vi "SetTriggerDelay.vi"(8 "error in (no error)":errorcluster, 10 "Arg":string, 11 "PCO in":refnum<class "PCO_Camera.lvclass">) -> (0 "error out":errorcluster, 2 "setValue out":dbl, 3 "PCO out":refnum<class "PCO_Camera.lvclass">)   [LabVIEW 2020, in "PCO_Camera.lvclass"]
uses:
  PCO_Camera.lvclass
  PCO_Camera.lvclass/PCO_Camera.ctl
  pco.labview/pco.camera/Camera.lvclass
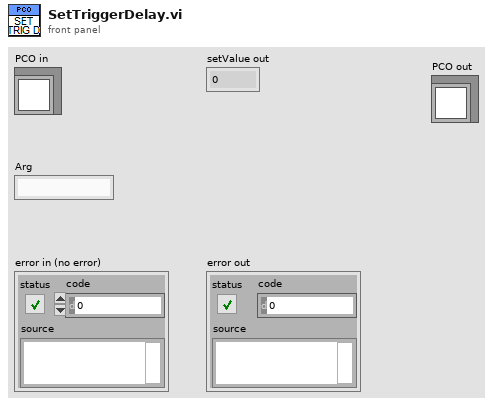
[diagram p1: front panel]
types:
  T1 = enum16{"sequence", "sequence non blocking", "ring buffer", "fifo", "sequence_dpcore", "sequence_non_blocking_dpcore", "ring_buffer_dpcore", "fifo_dpcore", "tif", "multitif", "pcoraw", "b16", "dicom", "multidicom"}
  T2 = typedef "Camera.lvclass/binning.ctl" = cluster{"vert":u16, "horz":u16}
  T3 = cluster{"exposure_time_s":dbl, "delay_time_s":dbl, "roi":cluster{"x0":u64, "y0":u64, "x1":u64, "y1":u64}, "timestamp_mode":u16, "pixelrate":u32, "trigger_mode":u16, "acquire_mode":u16, "metadata_mode":u16, "noisefilter_mode":u16, "binning":T2}
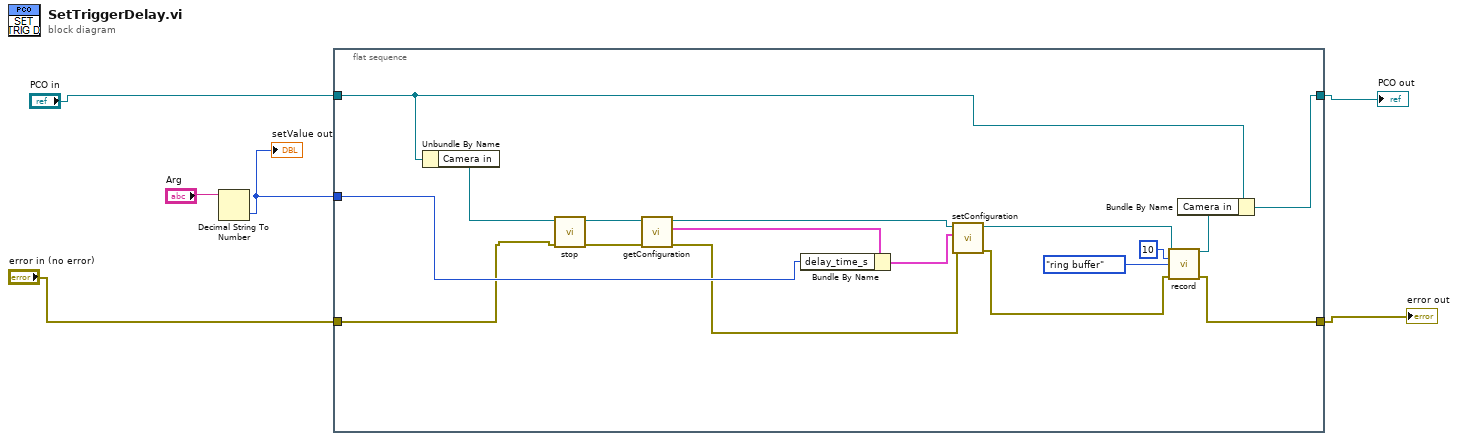
[diagram p0: block diagram]
diagram:
  n1 = Decimal String To Number(string="Arg") -> (number=w1:i32)  [unwired: 2 in, 1 out]
  "setValue out" <- w1
  n2 = flat-sequence {
    tunnel: "error in (no error)" -> [w14]
    tunnel: [w8] -> w4
    tunnel: "PCO in" -> [w23]
    tunnel: [w22] -> w2
    tunnel: w1 -> [w20]
    frame #0 {
      n3 = Unbundle By Name(w23) -> ("Camera in"=w16:refnum<class "Camera.lvclass">)
      n4 = call-dynamic "stop.vi"("error in (no error)"=w14, "Camera in"=w16) -> ("error out"=w13:errorcluster, "Camera out"=w15:refnum<class "Camera.lvclass">)  [unwired: 8 in]
      n5 = call-dynamic "getConfiguration.vi"("error in (no error)"=w13, "Camera in"=w15) -> ("error out"=w17:errorcluster, "configuration"=w21:T3, "Camera out"=w18:refnum<class "Camera.lvclass">)  [unwired: 7 in]
      n6 = Bundle By Name(cluster=w21, "delay_time_s"=w20) -> (w19:T3)
      n7 = call-dynamic "setConfiguration.vi"("error in (no error)"=w17, "configuration"=w19, "Camera in"=w18) -> ("error out"=w7:errorcluster, "Camera out"=w10:refnum<class "Camera.lvclass">)  [unwired: 7 in]
      n8 = call-dynamic "record.vi"("Camera in"=w10, "num_images"=u32 10, "record_mode"=T1."ring buffer", "error in (no error)"=w7) -> ("Camera out"=w9:refnum<class "Camera.lvclass">, "error out"=w8:errorcluster)  [unwired: 10 in]
      n9 = Bundle By Name(cluster=w23, "Camera in"=w9) -> (w22:refnum<class "PCO_Camera.lvclass">)
    }
  }
  "error out" <- w4
  "PCO out" <- w2
